vi "Main.vi"() -> ()   [LabVIEW 2026]
doc: "The Main VI of the Application. Responsible for the User interface of the application which involves catching user inputs and displaying the playfield."
uses:
  01_Typen/GameTetrominoInformationTypeDef.ctl
  01_Typen/GameCommandTypeDef.ctl
panel:
  in  "Stop VI":bool
  out "Game Over LED":bool caption="Game Over"
  in  "Move Left Button":bool
  in  "Rotate Button":bool
  in  "Move Right Button":bool
  in  "Reset Button":bool
  in  "Tetris Playfield":bool[][](array[boolean])
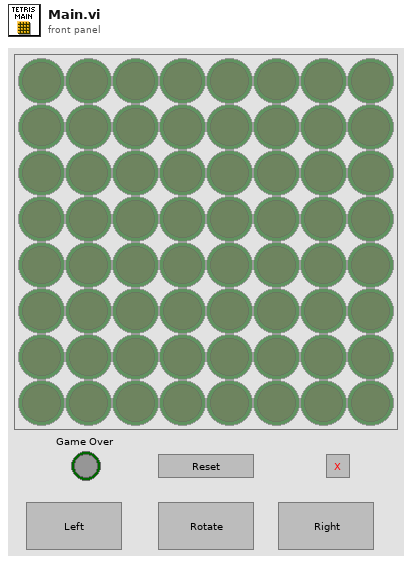
[diagram p1: front panel]
types:
  T1 = typedef "GameTetrominoInformationTypeDef.ctl" = cluster{"Block Position 1":cluster{"X":i32, "Y":i32}, "Block Position 2":cluster{"X":i32, "Y":i32}, "Block Position 3":cluster{"X":i32, "Y":i32}, "Block Position 4":cluster{"X":i32, "Y":i32}}
  T2 = typedef "GameCommandTypeDef.ctl" = enum16{"NoCommand", "Rotate", "MoveLeft", "MoveRight"}
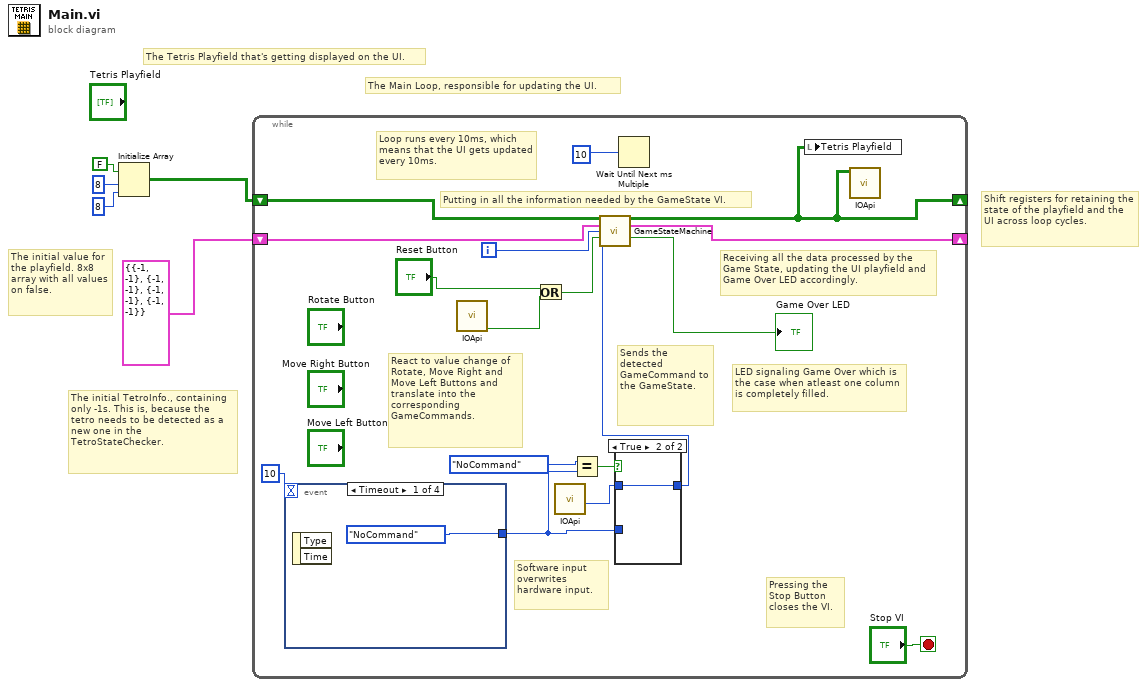
[diagram p0: block diagram]
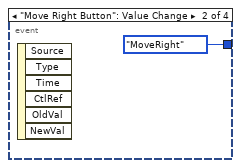
[diagram p3: hidden frame]
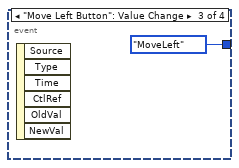
[diagram p4: hidden frame]
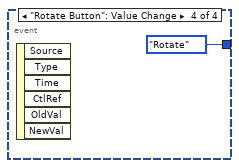
[diagram p5: hidden frame]
diagram:
  # "Shift registers for retaining the state of the playfield and the UI across loop cycles."
  # "The Main Loop, responsible for updating the UI."
  # "The Tetris Playfield that's getting displayed on the UI."
  # "The initial value for the playfield. 8x8 array with all values on false."
  # "The initial TetroInfo., containing only -1s. This is, because the tetro needs to be detected as a new one in the TetroStateChecker."
  n1 = Initialize Array(FALSE, 8 ("dimension size"), 8 ("dimension size")) -> (w2:bool[][])
  n2 = while {
    shift-right: [w14] -> _
    shift-left: w2 -> [w20]
    shift-right: [w16] -> _
    shift-left: T1 {"Block Position 1"={"X"=-1, "Y"=-1}, "Block Position 2"={"X"=-1, "Y"=-1}, "Block Position 3"={"X"=-1, "Y"=-1}, "Block Position 4"={"X"=-1, "Y"=-1}} ("Tile Info") -> [w17]
    i -> [w15]
    stop <- "Stop VI" stop-if-true
    # "Software input overwrites hardware input."
    # "Receiving all the data processed by the Game State, updating the UI playfield and Game Over LED accordingly."
    # "Putting in all the information needed by the GameState VI."
    # "LED signaling Game Over which is the case when atleast one column is completely filled."
    # "Sends the detected GameCommand to the GameState."
    # "Loop runs every 10ms, which means that the UI gets updated every 10ms."
    # "React to value change of Rotate, Move Right and Move Left Buttons and translate into the corresponding GameCommands."
    # "Pressing the Stop Button closes the VI."
    n3 = event shown="[0] Timeout" {
      selector: _ -> [_ _ _ _]
      dyn-events: _ -> [_ _ _ _]
      timeout: 10 -> [_ _ _ _]
      tunnel: [GameCommandTypeDef."NoCommand" ("Enum") GameCommandTypeDef."MoveRight" ("Enum") GameCommandTypeDef."MoveLeft" ("Enum") GameCommandTypeDef."Rotate" ("Enum")] -> w9
      event Timeout {
        n4 = event-data() -> ()  [unwired: 1 in, 2 out]
      }
      event "Move Right Button": Value Change {
        n5 = event-data() -> ()  [unwired: 1 in, 6 out]
      }
      event "Move Left Button": Value Change {
        n6 = event-data() -> ()  [unwired: 1 in, 6 out]
      }
      event "Rotate Button": Value Change {
        n7 = event-data() -> ()  [unwired: 1 in, 6 out]
      }
    }
    n8 = call "IOApi.vi"() -> ("Reset To Software"=w6:bool)  [unwired: 9 in, 2 out]
    n9 = Or(x="Reset Button", y=w6) -> (x .or. y?=w8:bool)
    n10 = call "IOApi.vi"() -> ("GameCommand To Software"=w12:T2)  [unwired: 9 in, 2 out]
    n11 = Equal?(x=GameCommandTypeDef."NoCommand" ("GameCommand enum"), y=w9) -> (x = y?=w13:bool)
    n12 = case shown="True" w13 {
      tunnel: w9 -> [w23 _]
      tunnel: w12 -> [_ w24]
      tunnel: [w23 w24] -> w11
      frame False {
      }
      frame True {
      }
    }
    n13 = call "GameStateMachine.vi"("Input Playfield"=w20, "Tile Info Input"=w17, "Loop iterator"=w15, "Input Reset"=w8, "Enum"=w11) -> ("Output Playfield"=w14:bool[][], "Tile Info Output"=w16:T1, "Game over"=→"Game Over LED":bool)  [unwired: 8 in]
    n14 = Wait Until Next ms Multiple(millisecond multiple=u32 10) -> ()  [unwired: 1 out]
    n15 = local write "Tetris Playfield"(w14) -> ()
    n16 = call "IOApi.vi"("Playfield From Software"=w14) -> ()  [unwired: 8 in, 3 out]
  }
